vi "Crate information.vi"(6 "code":i32, 7 "Status":bool, 8 "error in (no error)":errorcluster caption="错误输入（无错误）", 9 "Suroce":string, 10 "Type":enum16{"Inform", "Warning", "Alarm"}(ring), 11 "cause":string) -> (0 "error out":errorcluster caption="错误输出", 1 "appended array":string[](array[string]), 2 "Log Array":string[](array[string]), 3 "Log imform":string)   [LabVIEW 2014]
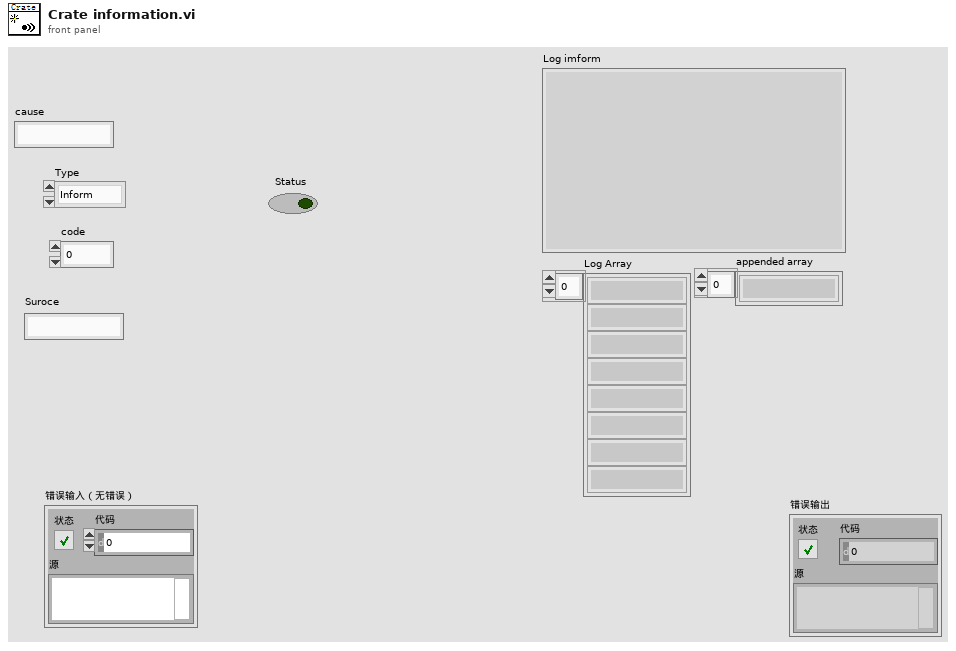
[diagram p1: front panel]
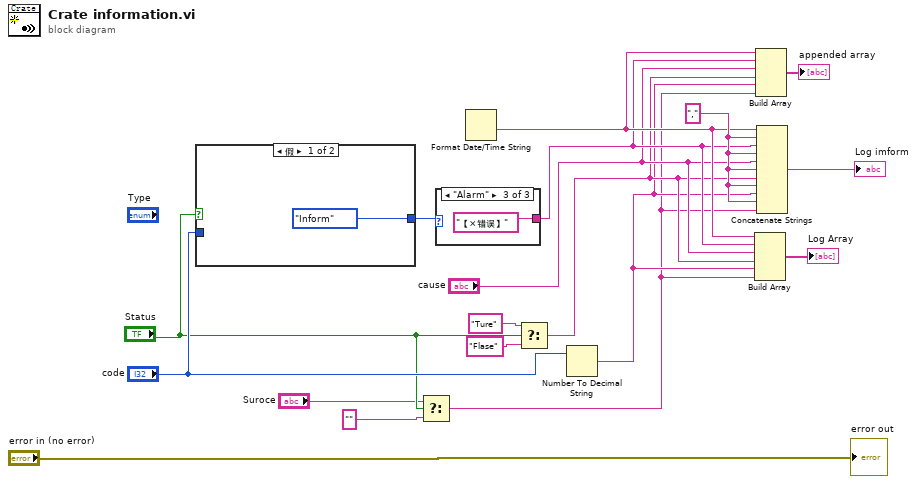
[diagram p0: block diagram]
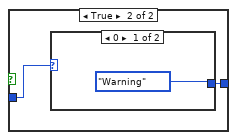
[diagram p2: hidden frame]
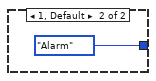
[diagram p3: hidden frame]
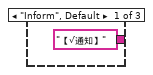
[diagram p4: hidden frame]
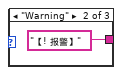
[diagram p5: hidden frame]
diagram:
  w13 = ","
  n1 = case shown="假" "Status" {
    tunnel: [enum16{"Inform", "Warning", "Alarm"}."Inform" ("Type") w20] -> w12
    tunnel: "code" -> [_ w21]
    frame False {
    }
    frame True {
      n2 = case shown="0" w21 {
        tunnel: [enum16{"Inform", "Warning", "Alarm"}."Warning" ("Type") enum16{"Inform", "Warning", "Alarm"}."Alarm" ("Type")] -> w20
        frame 0 {
        }
        frame 1, Default {
        }
      }
    }
  }
  n3 = Select(t="Suroce", s="Status", f="") -> (s? t:f=w2:string)
  n4 = case shown="\"Alarm\"" w12 {
    tunnel: ["【√通知】" ("时间格式字符串(%c)") "【! 报警】" ("时间格式字符串(%c)") "【×错误】" ("时间格式字符串(%c)")] -> w6
    frame "Inform", Default {
    }
    frame "Warning" {
    }
    frame "Alarm" {
    }
  }
  n5 = Format Date/Time String() -> (date/time string=w7:string)  [unwired: 3 in]
  n6 = Select(t="Ture", s="Status", f="Flase") -> (s? t:f=w4:string)
  n7 = Number To Decimal String(number="code") -> (decimal integer string=w3:string)  [unwired: 1 in]
  n8 = Build Array(w7, w6, "cause", w4, w3, w2) -> (→"Log Array":string[])
  n9 = Build Array(w7, w6, "cause", w4, w3, w2) -> (→"appended array":string[])
  n10 = Concatenate Strings(w7, w13, w6, w13, "cause", w13, w4, w13, w3, w13, w2) -> (→"Log imform":string)
  "error out" <- "error in (no error)"
